vi "Save MC data original.vi"(6 "Stop":bool, 7 "Initialise":bool, 8 "error in (no error)":errorcluster, 11 "Input":dbl[](array[numeric])) -> (0 "error out":errorcluster, 3 "MC Data Save ON":bool)   [LabVIEW 2020]
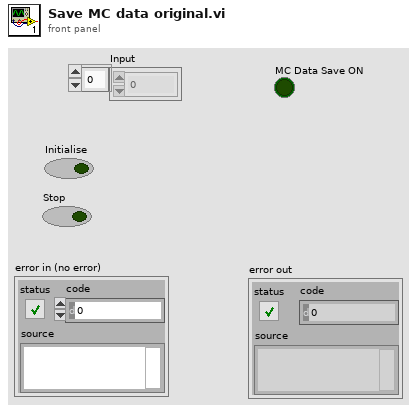
[diagram p1: front panel]
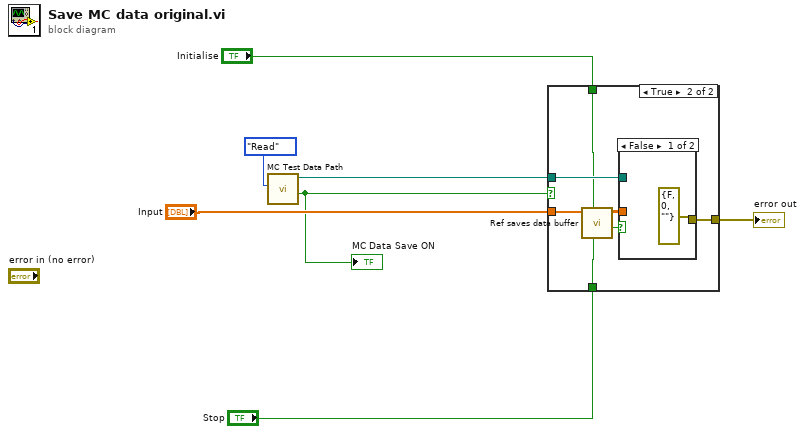
[diagram p0: block diagram]
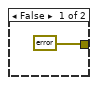
[diagram p2: hidden frame]
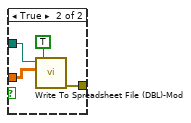
[diagram p3: hidden frame]
diagram:
  n1 = call "MC Test Data Path.vi"("State"=enum16{"Initialise", "Write", "Read"}."Read") -> ("Save Test Data"=w1:bool, "Test GraphData Path"=w6:path)  [unwired: 8 in, 1 out]
  "MC Data Save ON" <- w1
  n2 = case shown="True" w1 {
    tunnel: w6 -> [_ w15]
    tunnel: [errorcluster {"status"=FALSE, "code"=0, "source"=""} ("error out") w14] -> w5
    tunnel: "Input" -> [_ w13]
    tunnel: "Initialise" -> [_ w11]
    tunnel: "Stop" -> [_ w10]
    frame False {
    }
    frame True {
      n3 = call "Ref saves data buffer.vi"("Stop"=w10, "Initialise"=w11, "Array in"=w13) -> ("Save data"=w9:bool, "Array out"=w12:dbl[][])  [unwired: 7 in]
      n4 = case shown="False" w9 {
        tunnel: w15 -> [_ w20]
        tunnel: [errorcluster {"status"=FALSE, "code"=0, "source"=""} ("error out") w18] -> w14
        tunnel: w12 -> [_ w17]
        frame False {
        }
        frame True {
          n5 = call <userlib>:"Write To Spreadsheet File (DBL)-Mod.vi"("append to file? (new file:F)"=TRUE, "2D data"=w17, "file path (dialog if empty)"=w20) -> ("error out"=w18:errorcluster)  [unwired: 7 in, 1 out]
        }
      }
    }
  }
  "error out" <- w5
